vi "Load SPE v0.2.vi"(8 "Error In":errorcluster, 11 "File Path In":path) -> (0 "Error Out":errorcluster, 1 "DataBlock Info":T1, 2 "Output Stack":cluster{u16[][][]}[](array[cluster]), 3 "File Path Out":path, 4 "Parse Errors":string)   [LabVIEW 2012]
panel:
  out "Odd":bool
  out "XML Location":u64
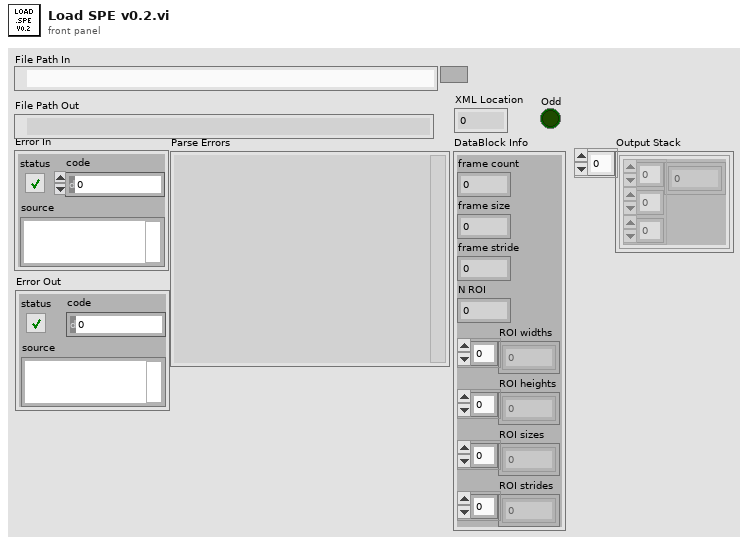
[diagram p1: front panel]
types:
  T1 = cluster{"frame count":i64, "frame size":i64, "frame stride":i64, "N ROI":i64, "ROI widths":i64[], "ROI heights":i64[], "ROI sizes":i64[], "ROI strides":i64[]}
  T2 = enum16{"open", "replace", "create", "open or create", "replace or create", "replace or create with confirmation"}
  T3 = enum16{"big-endian, network order", "native, host order", "little-endian"}
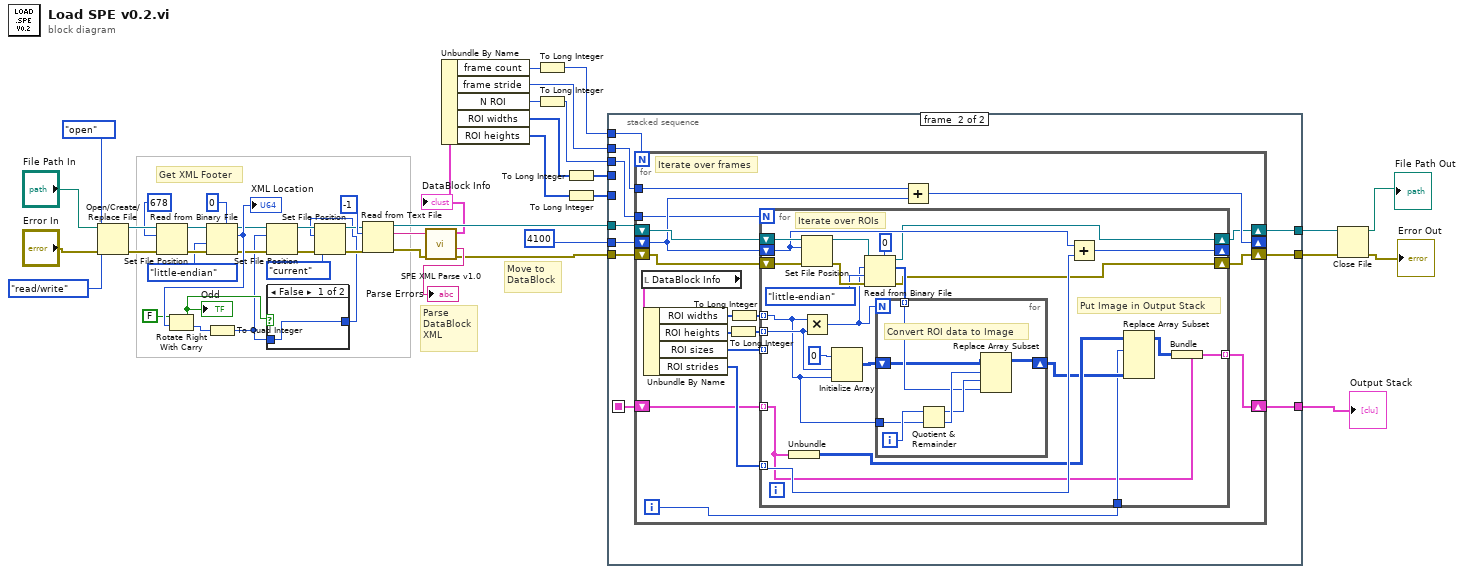
[diagram p0: block diagram]
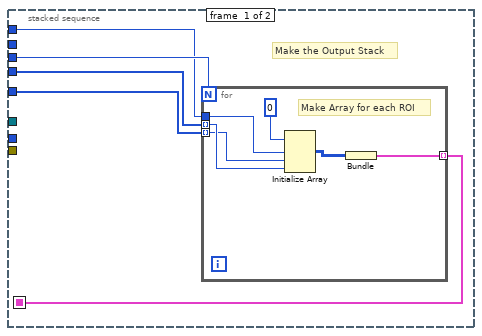
[diagram p2: hidden frame]
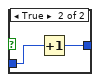
[diagram p3: hidden frame]
diagram:
  # "Parse\nDataBlock\nXML"
  # "Move to\nDataBlock"
  # "Get XML Footer"
  n1 = Open/Create/Replace File(file path (use dialog)="File Path In", error in="Error In", operation (0:open)=T2."open", access (0:read/write)=enum16{"read/write", "read-only", "write-only"}."read/write") -> (refnum out=w42:refnum<file>, error out=w43:errorcluster)  [unwired: 2 in, 1 out]
  n2 = Set File Position(offset (in bytes) (0)=i64 678, refnum=w42, error in=w43) -> (refnum out=w39:refnum<file>, error out=w40:errorcluster)  [unwired: 1 in]
  n3 = Read from Binary File(5:u64 0, 8:w40, 9:T3."little-endian" ("byte order (0:big-endian, network order)"), 11:w39) -> (0:w34:errorcluster, 2:w36:u64, 3:w33:refnum<file>)  [unwired: 2 in, 1 out]
  "XML Location" <- w36
  n4 = Rotate Right With Carry(2:w36, 3:FALSE ("carry")) -> (0:w32:u64, 1:w25:bool)
  "Odd" <- w25
  n5 = To Quad Integer(1:w32) -> (0:w3:i64)
  n6 = Set File Position(offset (in bytes) (0)=w3, refnum=w33, error in=w34) -> (refnum out=w29:refnum<file>, error out=w28:errorcluster)  [unwired: 1 in]
  n7 = case shown="False" w25 {
    tunnel: w3 -> [w47 w49]
    tunnel: [w47 w48] -> w26
    frame False {
    }
    frame True {
      n8 = Increment(x=w49) -> (x+1=w48:i64)
    }
  }
  n9 = Set File Position(offset (in bytes) (0)=w26, refnum=w29, from (0:start)=enum16{"start", "end", "current"}."current", error in=w28) -> (refnum out=w30:refnum<file>, error out=w31:errorcluster)
  n10 = Read from Text File(file (use dialog)=w30, count=-1, error in=w31) -> (refnum out=w24:refnum<file>, text=w21:string, error out=w22:errorcluster)  [unwired: 1 in, 1 out]
  n11 = call "SPE XML Parse v1.0.vi"("Error In"=w22, "XML String"=w21) -> ("Error Out"=w19:errorcluster, "Parse Errors"=→"Parse Errors":string, "DataBlock Info"=w18:T1)  [unwired: 6 in]
  "DataBlock Info" <- w18
  n12 = Unbundle By Name(w18) -> ("frame count"=w16:i64, "frame stride"=w15:i64, "N ROI"=w13:i64, "ROI widths"=w12:i64[], "ROI heights"=w11:i64[])
  n13 = To Long Integer(number=w16) -> (32bit integer=w17:i32)
  n14 = To Long Integer(number=w13) -> (32bit integer=w14:i32)
  n15 = To Long Integer(number=w12) -> (32bit integer=w10:i32[])
  n16 = To Long Integer(number=w11) -> (32bit integer=w9:i32[])
  n17 = stacked-sequence {
    seq-local: [w50 _] -> [_ w64]
    tunnel: w24 -> [_ w70]
    tunnel: i64 4100 ("offset (in bytes) (0)") -> [_ w69]
    tunnel: w19 -> [_ w68]
    tunnel: w17 -> [w51 w67]
    tunnel: w15 -> [_ w66]
    tunnel: w14 -> [w54 w65]
    tunnel: w10 -> [w53 _]
    tunnel: w9 -> [w52 _]
    tunnel: [_ w63] -> w6
    tunnel: [_ w62] -> w7
    tunnel: [_ w61] -> w8
    frame #0 {
      # "Make the Output Stack"
      n18 = for {
        N: w54 -> [_]
        tunnel: w53 -> [w58] mode=indexing
        tunnel: w52 -> [w57] mode=indexing
        tunnel: w51 -> [w59]
        tunnel: [w55] -> w50 mode=indexing
        # "Make Array for each ROI"
        n19 = Initialize Array(u16 0, w59, w57, w58) -> (w56:u16[][][])
        n20 = Bundle(w56) -> (w55:cluster{u16[][][]})  [unwired: 1 in]
      }
    }
    frame #1 {
      n21 = for {
        N: w67 -> [_]
        shift-right: [w84] -> w62
        shift-left: w70 -> [w87]
        shift-right: [w83] -> w63
        shift-left: w68 -> [w85]
        shift-right: [w88] -> _
        shift-left: w69 -> [w86]
        tunnel: w66 -> [w82]
        tunnel: w65 -> [w81]
        shift-right: [w71] -> w61
        shift-left: w64 -> [w73]
        i -> [w72]
        # "Iterate over frames"
        n22 = local read "DataBlock Info"() -> (w80:T1)
        n23 = Unbundle By Name(w80) -> ("ROI widths"=w79:i64[], "ROI heights"=w77:i64[], "ROI sizes"=w74:i64[], "ROI strides"=w75:i64[])
        n24 = To Long Integer(number=w77) -> (32bit integer=w76:i32[])
        n25 = To Long Integer(number=w79) -> (32bit integer=w78:i32[])
        n26 = for {
          N: w81 -> [_]
          shift-right: [w103] -> w84
          shift-left: w87 -> [w111]
          shift-right: [w105] -> _
          shift-left: w86 -> [w104]
          shift-right: [w97] -> w83
          shift-left: w85 -> [w110]
          tunnel: w78 -> [w95] mode=indexing
          tunnel: w76 -> [w96] mode=indexing
          tunnel: w75 -> [w101] mode=indexing
          tunnel: w74 -> [_] mode=indexing
          tunnel: w73 -> [w90] mode=indexing
          tunnel: w72 -> [w92]
          tunnel: [w89] -> w71 mode=indexing
          # "Put Image in Output Stack"
          # "Iterate over ROIs"
          n27 = Unbundle(w90) -> (w94:u16[][][])
          n28 = Set File Position(offset (in bytes) (0)=w104, refnum=w111, error in=w110) -> (refnum out=w109:refnum<file>, error out=w108:errorcluster)  [unwired: 1 in]
          n29 = Multiply(x=w95, y=w96) -> (x*y=w98:i32)
          n30 = Initialize Array(u16 0 ("element"), w96, w95) -> (w99:u16[][])
          n31 = Read from Binary File(5:u16 0, 8:w108, 9:T3."little-endian" ("byte order (0:big-endian, network order)"), 10:w98, 11:w109) -> (0:w97:errorcluster, 2:w102:u16[], 3:w103:refnum<file>)  [unwired: 1 in, 1 out]
          n32 = for {
            N: w98 -> [_]
            tunnel: w102 -> [w115] mode=indexing
            shift-right: [w114] -> w93
            shift-left: w99 -> [w112]
            tunnel: w95 -> [w113]
            i -> [w118]
            # "Convert ROI data to Image"
            n33 = Quotient & Remainder(x=w118, y=w113) -> (x-y*floor(x/y)=w116:i32, floor(x/y)=w117:i32)
            n34 = Replace Array Subset(array=w112, new element=w115, index (row)=w117, index (col)=w116) -> (w114:u16[][])
          }
          n35 = Add(x=w104, y=w101) -> (x+y=w105:i64)
          n36 = Replace Array Subset(array=w94, new element=w93, index (dim 0)=w92) -> (w91:u16[][][])  [unwired: 2 in]
          n37 = Bundle(cluster=w90, w91) -> (w89:cluster{u16[][][]})
        }
        n38 = Add(x=w82, y=w86) -> (x+y=w88:i64)
      }
    }
  }
  "Output Stack" <- w8
  n39 = Close File(refnum=w7, error in=w6) -> (path=→"File Path Out":path, error out=→"Error Out":errorcluster)
